vi "Contour Defect Inspection.vi"() -> ()   [LabVIEW 2014]
doc: "This example shows a contour analysis application. The contour of the rim of the can is extracted and a circle is fitted to those points. Then the contour is compared to the fitted circle to locate defects."
uses:
  <vilib>/vision/NI_Vision_Development_Module.lvlib
panel:
  out "Pass Status":bool
  in  "Max Distance":dbl=4.0 min=0.0 format="%.2f"
  out "Distance":dbl[](graph) caption="Distance of Contour from Fitted Circle"
  in  "Stop":bool
  out "Image":T1(plugin-control)
  in  "Delay (s.)":dbl(slide)=0.995260663507109 scale=0.0..3.0
  # "Overview: Demonstrates how to use the IMAQ Fit Contour function to compare the extracted contour against an expected shape contour and IMAQ Compute Contour Distance calculates the distance of the contour points from the expected shape.\nRequirements: Vision Development Software.\nInstructions:\n1. Run the VI.\n2. Adjust the Max Distance to change the distance tolerance. The locations that are greater than this maximum distance are overlaid in red on the image."
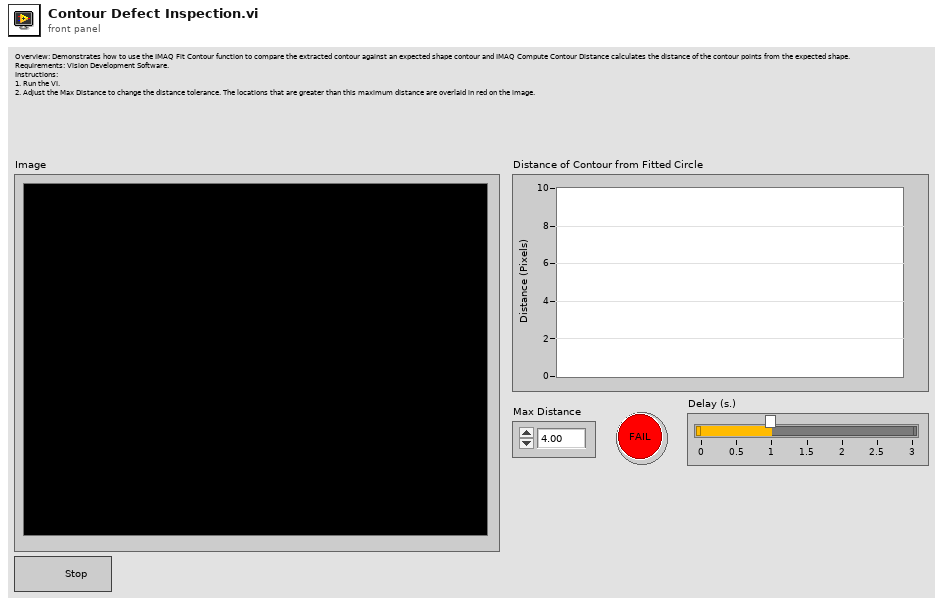
[diagram p1: front panel]
types:
  T1 = typedef "IMAQ Image.ctl" = refnum<image>
  T2 = typedef "IMAQ Circle" = cluster{"Center X":i32, "Center Y":i32, "Inner Radius":i32, "Outer Radius":i32, "Start Angle":dbl, "End Angle":dbl}
  T3 = typedef "ROI Descriptor" = cluster{"Global Rectangle":i32[], "Contours":cluster{"ID":enum32{"External", "Internal"}, "Type":u32, "Coordinates":i32[]}[]}
  T4 = cluster{"Overlay?":bool, "Color":u32, "Width":u32, "Maintain Width?":bool}
  T5 = enum16{"Closest To Search Start", "Maximum Length", "Strongest Mean Gradient Change"}
  T6 = enum16{"Rect Left To Right", "Rect Right To Left", "Rect Top To Bottom", "Rect Bottom To Top", "Annulus Inner To Outer", "Annulus Outer To Inner", "Annulus Start Angle To End Angle", "Annulus End Angle To Start Angle"}
  T7 = cluster{"Target Point":cluster{"X":dbl, "Y":dbl}, "Template Point":cluster{"X":dbl, "Y":dbl}, "Distance":dbl}[]
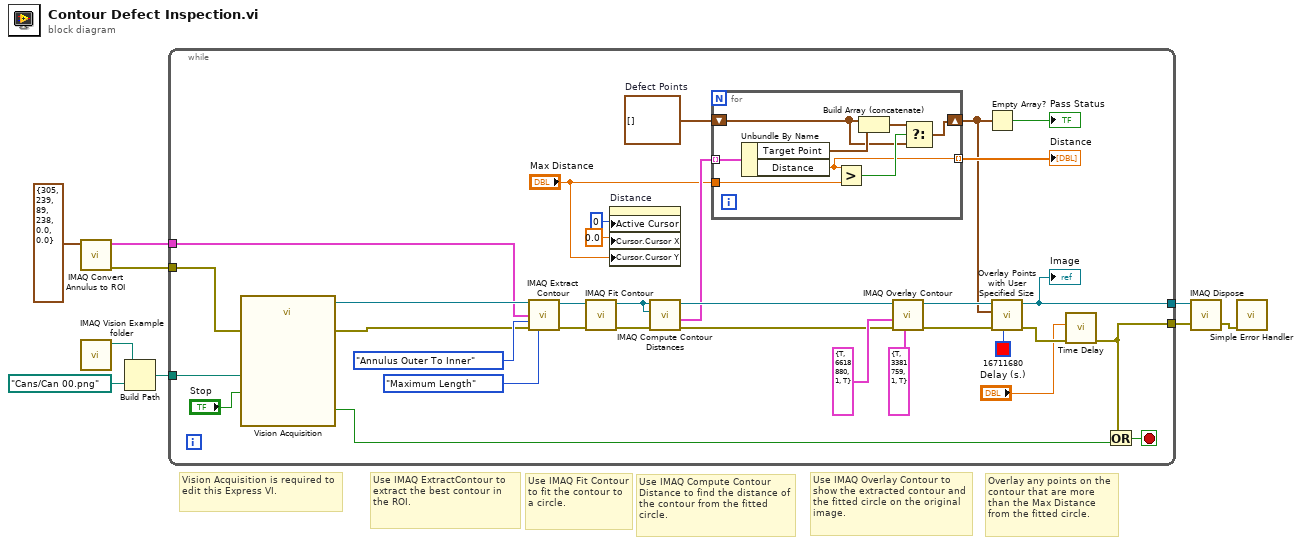
[diagram p0: block diagram]
diagram:
  # "Vision Acquisition is required to edit this Express VI."
  # "Overlay any points on the contour that are more than the Max Distance from the fitted circle."
  # "Use IMAQ Compute Contour Distance to find the distance of the contour from the fitted circle."
  # "Use IMAQ Fit Contour to fit the contour to a circle."
  # "Use IMAQ Overlay Contour to show the extracted contour and the fitted circle on the original image."
  # "Use IMAQ ExtractContour to extract the best contour in the ROI."
  n1 = call "IMAQ Convert Annulus to ROI"("Annulus"=T2 {"Center X"=305, "Center Y"=239, "Inner Radius"=89, "Outer Radius"=238, "Start Angle"=0.0, "End Angle"=0.0}) -> ("error out"=w1:errorcluster, "ROI Descriptor"=w4:T3)  [unwired: 8 in]
  n2 = call "IMAQ Vision Example folder.vi"() -> ("Example Image Path"=w6:path)  [unwired: 11 in]
  n3 = Build Path(base path=w6, name or relative path=path "Cans/Can 00.png") -> (appended path=w7:path)
  n4 = while {
    tunnel: [w26] -> w9
    tunnel: w7 -> [w23]
    tunnel: w4 -> [w22]
    tunnel: [w12] -> w3
    tunnel: w1 -> [w13]
    stop <- w11 stop-if-true
    w29 = cluster{"X":dbl, "Y":dbl}[] []  # Defect Points
    n5 = call "Vision Acquisition"("Image Path"=w23, "Stop (F)"="Stop", "error in"=w13) -> ("Image Out"=w25:T1, "Stopped"=w10:bool, "error out"=w24:errorcluster)  [unwired: 22 in]
    n6 = call "IMAQ Extract Contour"("Source Image"=w25, "ROI Descriptor"=w22, "Search Direction"=T6."Annulus Outer To Inner", "error in (no error)"=w24, "Contour Selection"=T5."Maximum Length") -> ("Source Image Out"=w35:T1, "error out"=w34:errorcluster)  [unwired: 3 in, 6 out]
    n7 = call-poly "IMAQ Fit Contour"("error in (no error)"=w34, "Contour Image"=w35) -> ("error out"=w40:errorcluster, "Contour Image Out"=w31:T1)  [unwired: 2 in, 6 out]
    n8 = property on="Distance" class="WFGraph (strict)"("Active Cursor"=u32 0, "Cursor.Cursor X"=0.0 ("Cursor.Cursor Position:Cursor X"), "Cursor.Cursor Y"="Max Distance") -> ()  [unwired: 2 in, 2 out]
    n9 = call "IMAQ Compute Contour Distances"("error in (no error)"=w40, "Template Contour Image"=w31, "Target Contour Image"=w31) -> ("error out"=w36:errorcluster, "Distances"=w30:T7, "Target Contour Image Out (dup)"=w37:T1)  [unwired: 2 in, 4 out]
    n10 = for {
      tunnel: w30 -> [w50] mode=indexing
      shift-right: [w45] -> w20
      shift-left: w29 -> [w46]
      tunnel: [w44] -> w21 mode=indexing
      tunnel: "Max Distance" -> [w43]
      n11 = Unbundle By Name(w50) -> ("Target Point"=w49:cluster{"X":dbl, "Y":dbl}, "Distance"=w44:dbl)
      n12 = Greater?(x=w44, y=w43) -> (0:w48:bool)
      n13 = Build Array (concatenate)(w46, w49) -> (w47:cluster{"X":dbl, "Y":dbl}[])
      n14 = Select(t=w47, s=w48, f=w46) -> (s? t:f=w45:cluster{"X":dbl, "Y":dbl}[])
    }
    "Distance" <- w21
    n15 = call "IMAQ Overlay Contour"("Contour Equation Settings"=T4 {"Overlay?"=TRUE, "Color"=3381759, "Width"=1, "Maintain Width?"=TRUE}, "error in (no error)"=w36, "Contour Points Settings"=T4 {"Overlay?"=TRUE, "Color"=6618880, "Width"=1, "Maintain Width?"=TRUE}, "Image"=w37) -> ("error out"=w14:errorcluster, "Image Out"=w28:T1)  [unwired: 2 in, 4 out]
    n16 = Empty Array?(array=w20) -> (empty?=→"Pass Status":bool)
    n17 = call "Overlay Points with User Specified Size.vi"("Color"=u32 16711680, "error in"=w14, "Points"=w20, "Image In"=w28) -> ("error out"=w16:errorcluster, "Image Out"=w26:T1)  [unwired: 6 in]
    "Image" <- w26
    n18 = call "Time Delay"("error in (no error)"=w16, "Delay Time (s)"="Delay (s.)") -> ("error out"=w12:errorcluster)  [unwired: 9 in]
    n19 = Or(x=w12, y=w10) -> (x .or. y?=w11:bool)
  }
  n20 = call "IMAQ Dispose"("Image"=w9, "error in (no error)"=w3) -> ("error out"=w2:errorcluster)  [unwired: 1 in, 3 out]
  n21 = call <vilib>:"Simple Error Handler.vi"("error in (no error)"=w2) -> ()  [unwired: 4 in, 5 out]
